vi "mod_LDPC Calculate Likelihoods (AWGN).vi"(0 "input complex waveform":T1 {"Y" format="%.3f"; "dt" format="%^.2e"; "t0" format="%.4f"}, 5 "symbol map":cdb[](array[numeric]), 9 "sigma":dbl=0.3, 11 "error in (no error)":errorcluster) -> (4 "likelihoods out":dbl[](array[numeric]), 15 "error out":errorcluster)   [LabVIEW 2020, in "niDMT.lvlib"]
uses:
  <vilib>/addons/Modulation/niDMT.lvlib
  <vilib>/addons/Modulation/Analog/controls/Complex Data Waveform.ctl
  <vilib>/addons/Modulation/niAMT.lvlib
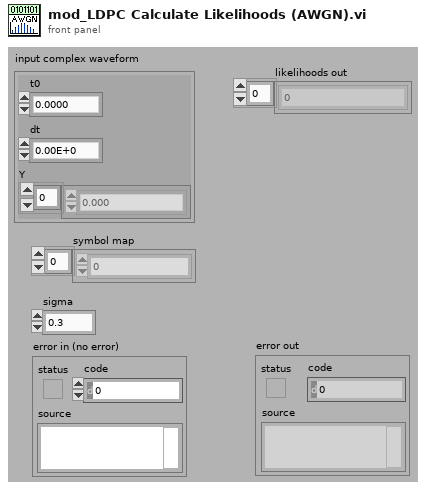
[diagram p1: front panel]
types:
  T1 = typedef "niAMT.lvlib/Complex Data Waveform.ctl" = cluster{"t0":dbl, "dt":dbl, "Y":cdb[]}
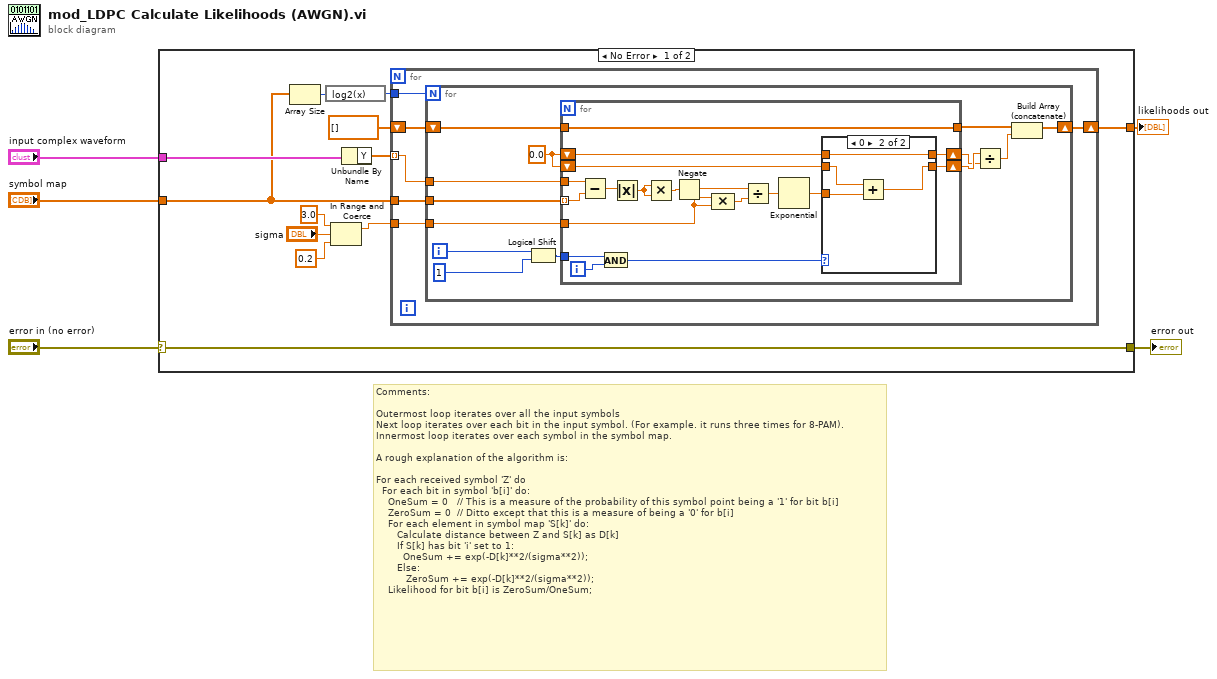
[diagram p0: block diagram]
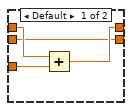
[diagram p2: hidden frame]
diagram:
  # "Comments:\n\nOutermost loop iterates over all the input symbols\nNext loop iterates over each bit in the input symbol. (For example. it runs three times for 8-PAM).\nInnermost loop iterates over each symbol in the symbol map.\n\nA rough explanation of the algorithm is:\n\nFor each received symbol 'Z' do\n  For each bit in symbol 'b[i]' do:\n    OneSum = 0   // This is a measure of the probability of this symbol point being a '1' for bit b[i]\n    ZeroSum = 0  // Ditto except that this is a measure of being a '0' for b[i]\n    For each element in symbol map 'S[k]' do:\n       Calculate distance between Z and S[k] as D[k]\n       If S[k] has bit 'i' set to 1:\n         OneSum += exp(-D[k]**2/(sigma**2));\n       Else:\n          ZeroSum += exp(-D[k]**2/(sigma**2));\n    Likelihood for bit b[i] is ZeroSum/OneSum;"
  n1 = case shown="No Error" "error in (no error)" {
    selector: "error in (no error)" -> [w11 w63]
    tunnel: "input complex waveform" -> [w17 _]
    tunnel: [w12 _] -> w3
    tunnel: [w11 w63] -> w2
    tunnel: "symbol map" -> [w10 _]
    frame No Error {
      n2 = Array Size(array=w10) -> (size(s)=w14:i32)
      n3 = expression code="log2(x)"(w14) -> (w13:i32)
      n4 = In Range and Coerce(upper limit=3.0, x="sigma", lower limit=0.2) -> (coerced(x)=w6:dbl)  [unwired: 1 out]
      n5 = Unbundle By Name(w17) -> ("Y"=w16:cdb[])
      n6 = for {
        tunnel: w16 -> [w20] mode=indexing
        shift-right: [w19] -> w12
        shift-left: dbl[] [] -> [w22]
        tunnel: w13 -> [w23]
        tunnel: w10 -> [w21]
        tunnel: w6 -> [w18]
        n7 = for {
          N: w23 -> [_]
          shift-right: [w26] -> w19
          shift-left: w22 -> [w32]
          tunnel: w21 -> [w35]
          tunnel: w20 -> [w31]
          tunnel: w18 -> [w24]
          i -> [w25]
          w34 = 0.0
          n8 = Logical Shift(y=w25, x=1) -> (x << y=w33:i32)
          n9 = for {
            tunnel: w35 -> [w51] mode=indexing
            shift-right: [w44] -> w29
            shift-left: w34 -> [w47]
            shift-right: [w43] -> w30
            shift-left: w34 -> [w46]
            tunnel: w33 -> [w53]
            tunnel: w31 -> [w52]
            tunnel: w32 -> [w42]
            tunnel: [w42] -> w27
            tunnel: w24 -> [w38]
            i -> [w54]
            n10 = Subtract(x=w52, y=w51) -> (x-y=w41:cdb)
            n11 = And(x=w53, y=w54) -> (x .and. y?=w48:i32)
            n12 = Absolute Value(x=w41) -> (abs(x)=w40:dbl)
            n13 = Multiply(x=w40, y=w40) -> (x*y=w39:dbl)
            n14 = Negate(x=w39) -> (-x=w37:dbl)
            n15 = Compound Arithmetic op=MULTIPLY(w38, w38) -> (w50:dbl)
            n16 = Divide(x=w37, y=w50) -> (x/y=w49:dbl)
            n17 = Exponential(1:w49) -> (0:w45:dbl)
            n18 = case shown="0" w48 {
              tunnel: w47 -> [w57 w61]
              tunnel: w46 -> [w55 w60]
              tunnel: w45 -> [w58 w62]
              tunnel: [w56 w61] -> w44
              tunnel: [w55 w59] -> w43
              frame Default {
                n19 = Add(x=w57, y=w58) -> (x+y=w56:dbl)
              }
              frame 0 {
                n20 = Add(x=w60, y=w62) -> (x+y=w59:dbl)
              }
            }
          }
          n21 = Divide(x=w30, y=w29) -> (x/y=w28:dbl)
          n22 = Build Array (concatenate)(w27, w28) -> (w26:dbl[])
        }
      }
    }
    frame Error {
    }
  }
  "likelihoods out" <- w3
  "error out" <- w2
